vi "状态改变.vi"(10 "附加信息":string, 11 "设备状态":enum16{"设备离线", "设备正常", "设备缺料", "设备故障", "质量报警"}(ring)=enum."设备缺料") -> ()   [LabVIEW 2018]
uses:
  Database/Global1.vi
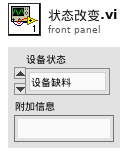
[diagram p1: front panel]
types:
  T1 = cluster{"用户编号":string, "用户名":string, "用户密码(密文)":string, "用户权限":string}
  T2 = cluster{"设备名称":string, "用户名":string, "设备状态":enum16{"设备离线", "设备正常", "设备缺料", "设备故障", "质量报警"}, "附加信息":string}
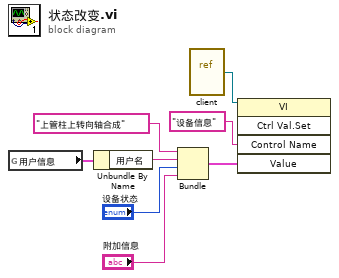
[diagram p0: block diagram]
diagram:
  n1 = global read "Global1.vi" "用户信息"() -> (w6:T1)
  n2 = Unbundle By Name(w6) -> ("用户名"=w4:string)
  n3 = Bundle("设备名称"="上管柱上转向轴合成", "用户名"=w4, "设备状态"="设备状态", "附加信息"="附加信息") -> (w1:T2)  [unwired: 1 in]
  n4 = vi-ref "client.vi"() -> (w8:refnum<vi>)
  n5 = invoke class="VI" method="Ctrl Val.Set"(reference=w8, "Control Name"="设备信息" ("控件名"), "Value"=w1) -> ()  [unwired: 2 in, 5 out]
